vi "loadData.vi"() -> ()   [LabVIEW 2014, in "SETI_LV.lvlib"]
uses:
  SETI_LV/SETI_LV.lvlib
  ChirpFFT Pairs.ctl
  Power Spectrum Data.ctl
  <vilib>/Analysis/2dsp.llb/Complex FFT.vi
  <vilib>/Analysis/NI_AALPro.lvlib
panel:
  out "Chirp/Fft Pair 1 - Chirp Rate":dbl
  out "Array":i32[](array[numeric])
  out "Chirp/Fft Pair 1 - Fft Length":i32
  out "Chirped Data":csg[](array[numeric])
  in  "error in":errorcluster
  in  "Max Error":dbl=0.0001 format="%#_6f"
  out "Number of Power Spectrums (from file)":i32
  out "Number of Chirp Pairs":i32
  out "Array of Greatest Error Less that 1E-5":bool[](array[boolean])
  out "Current icfft":i32
  out "Greatest Error Less that 1E-5":bool=TRUE
  out "Power Spectrum (from file)":sgl[](array[numeric])
  out "Error (greatest to smallest)":dbl[](array[numeric]) format="%#_6f"
  out "Power Spectrum Data":T1[](array[typedef])
  out "Power Spectrum":dbl[](array[numeric]) format="%_10g"
  out "FFT {X}":cdb[](array[numeric]) format="%_10g"
  out "d":sgl=-0.01266181
  out "c":sgl=0.99991983
  out "ang":dbl=1.9979847564988014
  out "time":dbl=26.84345694384995
  out "ChirpData":csg[](array[numeric]) format="%_8g"
  out "end_icfft":i32=20
  out "start_icfft":i32=16
  out "Chirp FFT Pairs":T2[](array[typedef])
  out "binWorkUnitDataPoints.bin (DataIn)":csg[](array[numeric])
  out "NumDataPoints":u32=262144
  out "error out":errorcluster
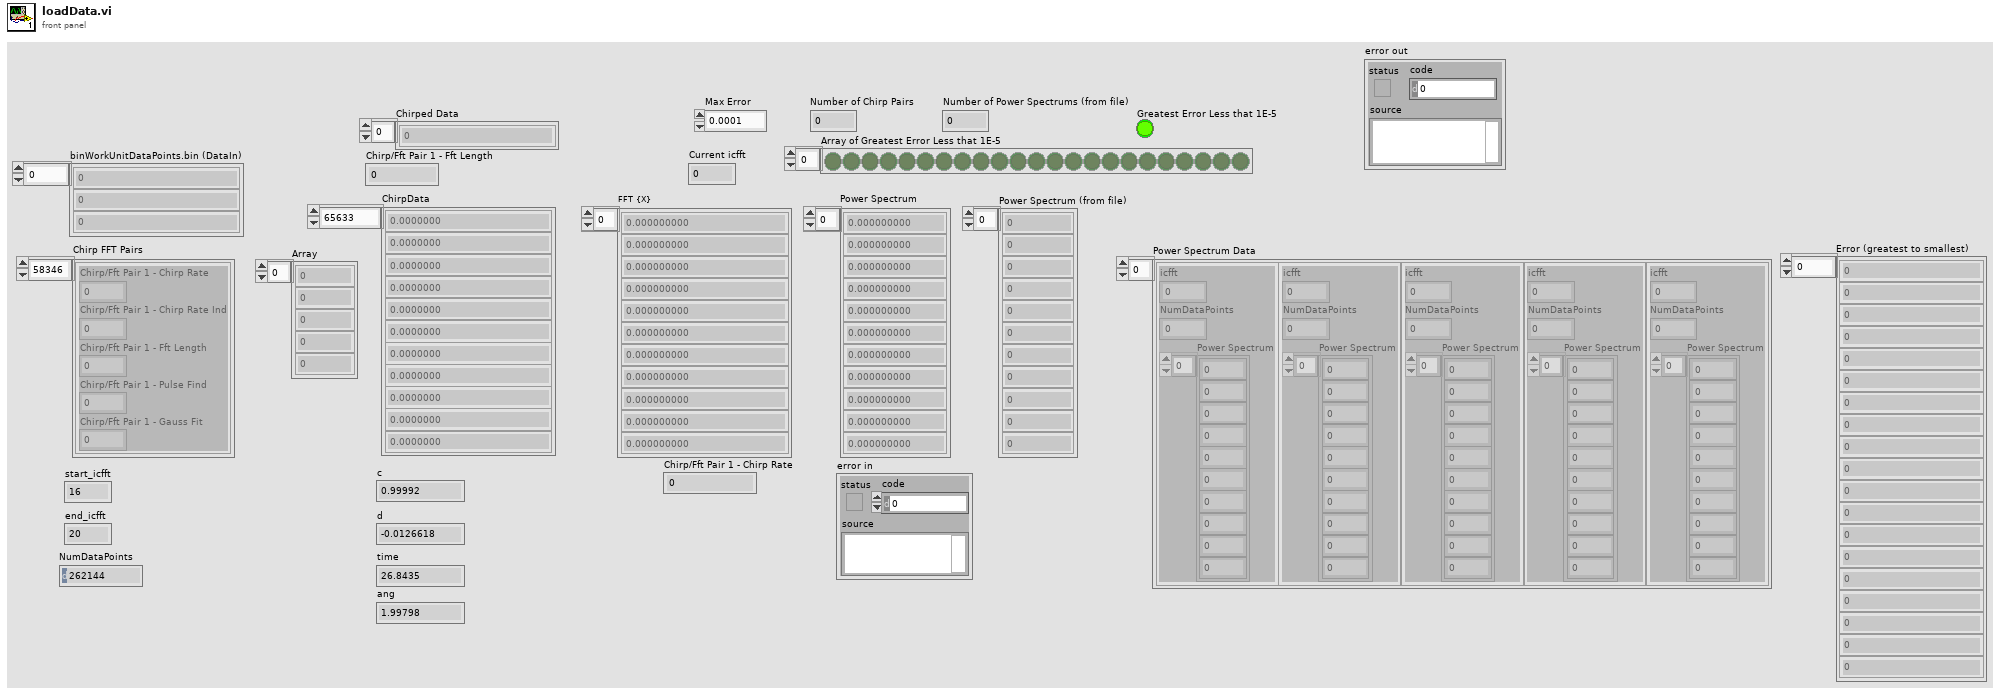
[diagram p1: front panel]
types:
  T1 = typedef "SETI_LV.lvlib/Power Spectrum Data.ctl" = cluster{"icfft":i32, "NumDataPoints":i32, "Power Spectrum":sgl[]}
  T2 = typedef "SETI_LV.lvlib/ChirpFFT Pairs.ctl" = cluster{"Chirp/Fft Pair 1 - Chirp Rate":dbl, "Chirp/Fft Pair 1 - Chirp Rate Ind":i32, "Chirp/Fft Pair 1 - Fft Length":i32, "Chirp/Fft Pair 1 - Pulse Find":i32, "Chirp/Fft Pair 1 - Gauss Fit":i32}
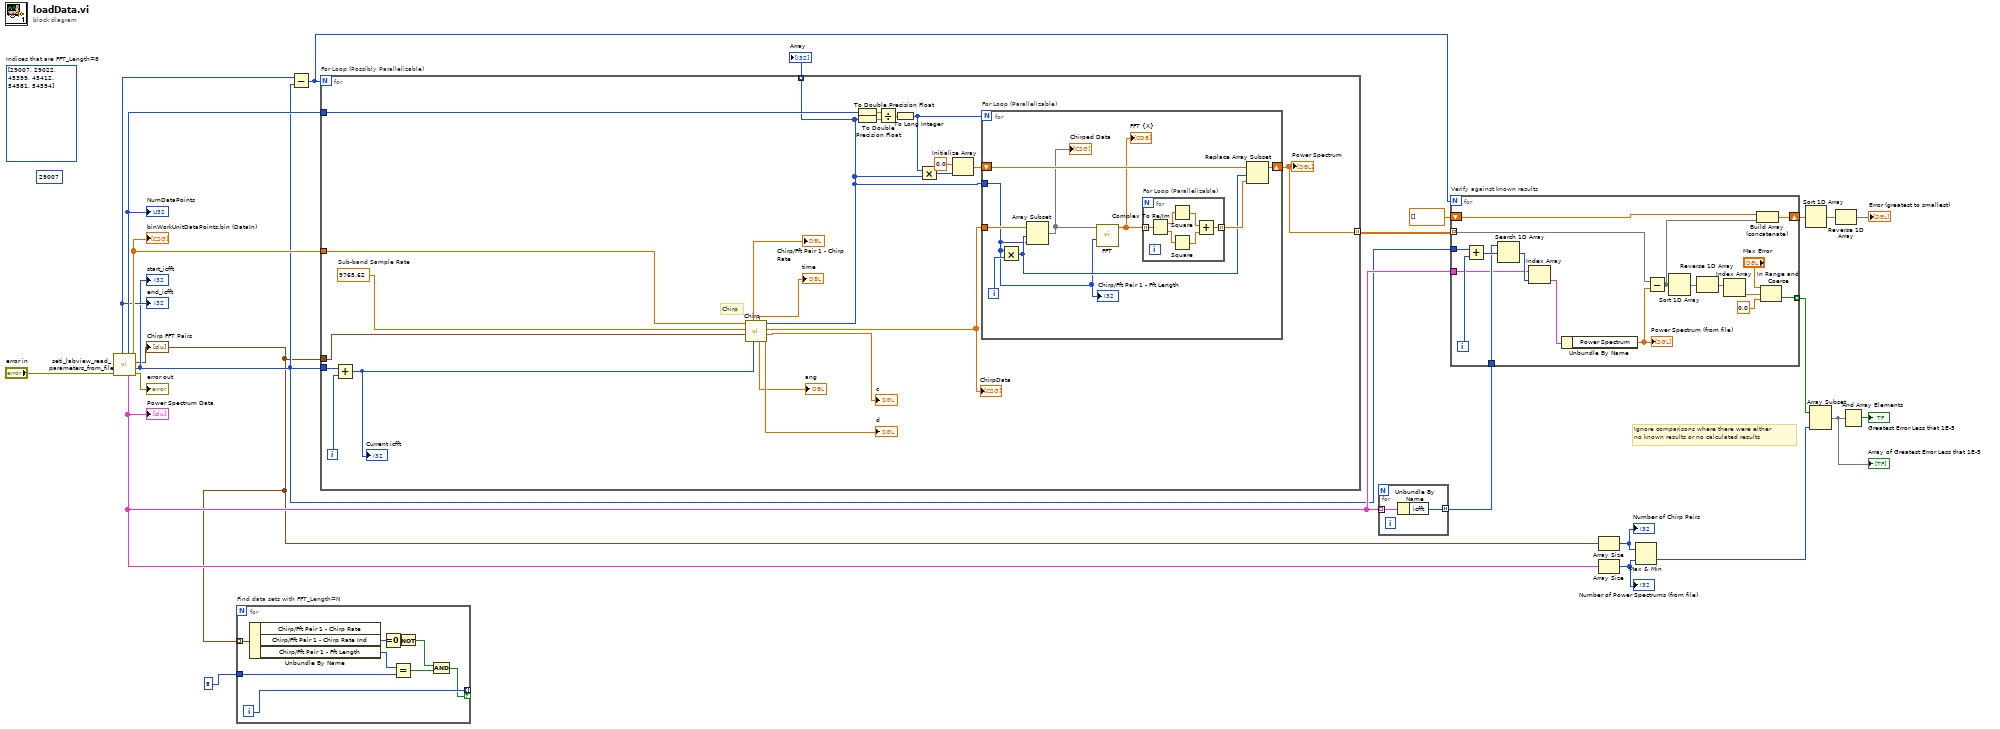
[diagram p0: block diagram]
diagram:
  (unwired) i32[] [29007, 29022, 45399, 45412, 54581, 54594]  # Indices that are FFT_Length=8
  (unwired) 29007 ("Numeric Control")
  # "Ignore comparisons where there were either\nno known results or no calculated results"
  n1 = call "seti_labview_read_parameters_from_file.vi"("error in (no error)"="error in") -> ("error out"=→"error out":errorcluster, "start_icfft"=w3:i32, "Chirp FFT Pairs"=w2:T2[], "binWorkUnitDataPoints.bin (DataIn)"=w23:csg[], "Array of Power Spectrum Data"=w10:T1[], "NumDataPoints"=w22:u32, "end_icfft"=w4:i32)  [unwired: 4 in]
  "NumDataPoints" <- w22
  "binWorkUnitDataPoints.bin (DataIn)" <- w23
  "Chirp FFT Pairs" <- w2
  "start_icfft" <- w3
  "end_icfft" <- w4
  "Power Spectrum Data" <- w10
  n2 = for "Find data sets with FFT_Length=N" {
    tunnel: w2 -> [w31] mode=indexing
    tunnel: [w26] -> _ mode=indexing if=w25
    tunnel: 8 ("y") -> [w24]
    i -> [w26]
    n3 = Unbundle By Name(w31) -> ("Chirp/Fft Pair 1 - Chirp Rate Ind"=w32:i32, "Chirp/Fft Pair 1 - Fft Length"=w29:i32)  [unwired: 1 out]
    n4 = Equal To 0?(x=w32) -> (x = 0?=w30:bool)
    n5 = Equal?(x=w29, y=w24) -> (x = y?=w27:bool)
    n6 = Not(x=w30) -> (.not. x?=w28:bool)
    n7 = And(x=w28, y=w27) -> (x .and. y?=w25:bool)
  }
  n8 = Subtract(x=w4, y=w3) -> (x-y=w14:i32)
  n9 = for "For Loop (Possibly Parallelizable)" {
    N: w14 -> [_]
    tunnel: w3 -> [w54]
    tunnel: w2 -> [w53]
    tunnel: w23 -> [w52]
    tunnel: w22 -> [w49]
    tunnel: [w39] -> w13 mode=indexing
    tunnel: [w38] -> w5 mode=indexing
    i -> [w46]
    w51 = 9765.62  # Sub-band Sample Rate
    # "Chirp"
    n10 = Add(x=w54, y=w46) -> (x+y=w37:i32)
    "Current icfft" <- w37
    n11 = call "Chirp"("icfft"=w37, "Chirp FFT Pairs"=w53, "Sub-band Sample Rate"=w51, "binWorkUnitDataPoints.bin (DataIn) in"=w52) -> ("d"=→"d":sgl, "c"=→"c":sgl, "binWorkUnitDataPoints.bin (DataIn) out"=w47:csg[], "Chirp/Fft Pair 1 - Fft Length"=w38:i32, "ang"=→"ang":dbl, "time"=→"time":dbl, "Chirp/Fft Pair 1 - Chirp Rate"=→"Chirp/Fft Pair 1 - Chirp Rate":dbl)  [unwired: 1 in]
    "ChirpData" <- w47
    n12 = To Double Precision Float(number=w49) -> (double precision float=w45:dbl)
    n13 = To Double Precision Float(number=w38) -> (double precision float=w44:dbl)
    n14 = Divide(x=w45, y=w44) -> (x/y=w48:dbl)
    n15 = To Long Integer(number=w48) -> (32bit integer=w40:i32)
    n16 = Multiply(x=w40, y=w38) -> (x*y=w41:i32)
    n17 = Initialize Array(0.0, w41) -> (w42:dbl[])
    n18 = for "For Loop (Parallelizable)" {
      N: w40 -> [_]
      tunnel: w47 -> [w63]
      tunnel: w38 -> [w56]
      shift-right: [w60] -> w39
      shift-left: w42 -> [w61]
      i -> [w62]
      n19 = Multiply(x=w56, y=w62) -> (x*y=w58:i32)
      n20 = Array Subset(array=w63, index=w58, length=w56) -> (w55:csg[])
      "Chirped Data" <- w55
      n21 = call-poly <vilib>:"FFT.vi"("FFT size"=w56, "X"=w55) -> ("FFT {X}"=w57:cdb[])  [unwired: 8 in, 1 out]
      "FFT {X}" <- w57
      n22 = for "For Loop (Parallelizable)" {
        tunnel: w57 -> [w69] mode=indexing
        tunnel: [w66] -> w59 mode=indexing
        n23 = Complex To Re/Im(x + iy=w69) -> (x=w68:dbl, y=w67:dbl)
        n24 = Square(x=w68) -> (x^2=w65:dbl)
        n25 = Square(x=w67) -> (x^2=w64:dbl)
        n26 = Add(x=w65, y=w64) -> (x+y=w66:dbl)
      }
      n27 = Replace Array Subset(array=w61, new element=w59, index=w58) -> (w60:dbl[])
      "Chirp/Fft Pair 1 - Fft Length" <- w56
    }
    "Power Spectrum" <- w39
  }
  "Array" <- w5
  n28 = for {
    tunnel: w10 -> [w71] mode=indexing
    tunnel: [w70] -> w12 mode=indexing
    n29 = Unbundle By Name(w71) -> ("icfft"=w70:i32)
  }
  n30 = for "Verify against known results" {
    N: w14 -> [_]
    tunnel: w13 -> [w75] mode=indexing
    tunnel: w3 -> [w88]
    tunnel: w12 -> [w85]
    tunnel: [w77] -> w11 mode=indexing
    tunnel: w10 -> [w76]
    shift-right: [w73] -> w8
    shift-left: dbl[] [] -> [w72]
    i -> [w87]
    n31 = Add(x=w88, y=w87) -> (x+y=w86:i32)
    n32 = Search 1D Array(1D array=w85, element=w86) -> (index of element=w89:i32)  [unwired: 1 in]
    n33 = Index Array(array=w76, index=w89) -> (element=w78:T1)
    n34 = Unbundle By Name(w78) -> ("Power Spectrum"=w80:sgl[])
    "Power Spectrum (from file)" <- w80
    n35 = Subtract(x=w75, y=w80) -> (x-y=w74:dbl[])
    n36 = Sort 1D Array(array=w74) -> (sorted array=w79:dbl[])
    n37 = Reverse 1D Array(array=w79) -> (reversed array=w81:dbl[])
    n38 = Index Array(array=w81) -> (element=w84:dbl)  [unwired: 1 in]
    n39 = Build Array (concatenate)(w72, w74) -> (w73:dbl[])
    n40 = In Range and Coerce(upper limit="Max Error", x=w84, lower limit=0.0) -> (In Range?=w77:bool)  [unwired: 1 out]
  }
  n41 = Array Size(array=w2) -> (size(s)=w19:i32)
  "Number of Chirp Pairs" <- w19
  n42 = Array Size(array=w10) -> (size(s)=w16:i32)
  "Number of Power Spectrums (from file)" <- w16
  n43 = Max & Min(x=w19, y=w16) -> (min(x,y)=w17:i32)  [unwired: 1 out]
  n44 = Sort 1D Array(array=w8) -> (sorted array=w9:dbl[])
  n45 = Array Subset(array=w11, length=w17) -> (w18:bool[])  [unwired: 1 in]
  "Array of Greatest Error Less that 1E-5" <- w18
  n46 = Reverse 1D Array(array=w9) -> (reversed array=→"Error (greatest to smallest)":dbl[])
  n47 = And Array Elements(Boolean array=w18) -> (logical AND=→"Greatest Error Less that 1E-5":bool)
